vi "ArmFF_MaxAchieveVelocity.vi"(8 "Acceleration":dbl, 9 "Angle":dbl, 10 "MaxVoltage":dbl, 11 "in ARM_FF":T1 {"kCos" format="%13.5p"; "Ka" format="%13.5p"; "Kv" format="%13.5p"; "Ks" format="%13.5p"}) -> (3 "MaxVelocity":dbl)   [LabVIEW 2019, in "Trajectory_Library.lvlib"]
doc: "Calculates the maximum achievable velocity given a maximum voltage supply, a position, and an acceleration. Useful for ensuring that velocity and acceleration constraints for a trapezoidal profile are simultaneously achievable - enter the acceleration constraint, and this will give you a simultaneously-achievable velocity constraint.\n \nInputs: \n - ArmFF -- The ArmFF data cluster\n - maxVoltage -- The maximum voltage that can be supplied to the arm.\n - angle -- The angle of the arm. (radians)\n - acceleration -- The acceleration of the arm.\n\nOutputs:\n - MaxVelocity -- The maximum possible velocity at the given acceleration and angle."
uses:
  Trajectory_Library.lvlib
  ARM_FF.ctl
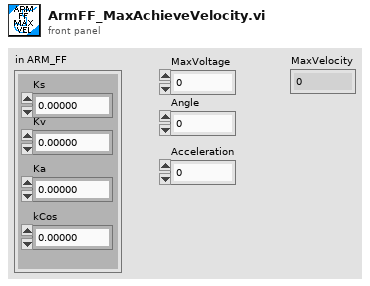
[diagram p1: front panel]
types:
  T1 = typedef "Trajectory_Library.lvlib/ARM_FF.ctl" = cluster{"Ks":dbl, "Kv":dbl, "Ka":dbl, "kCos":dbl}
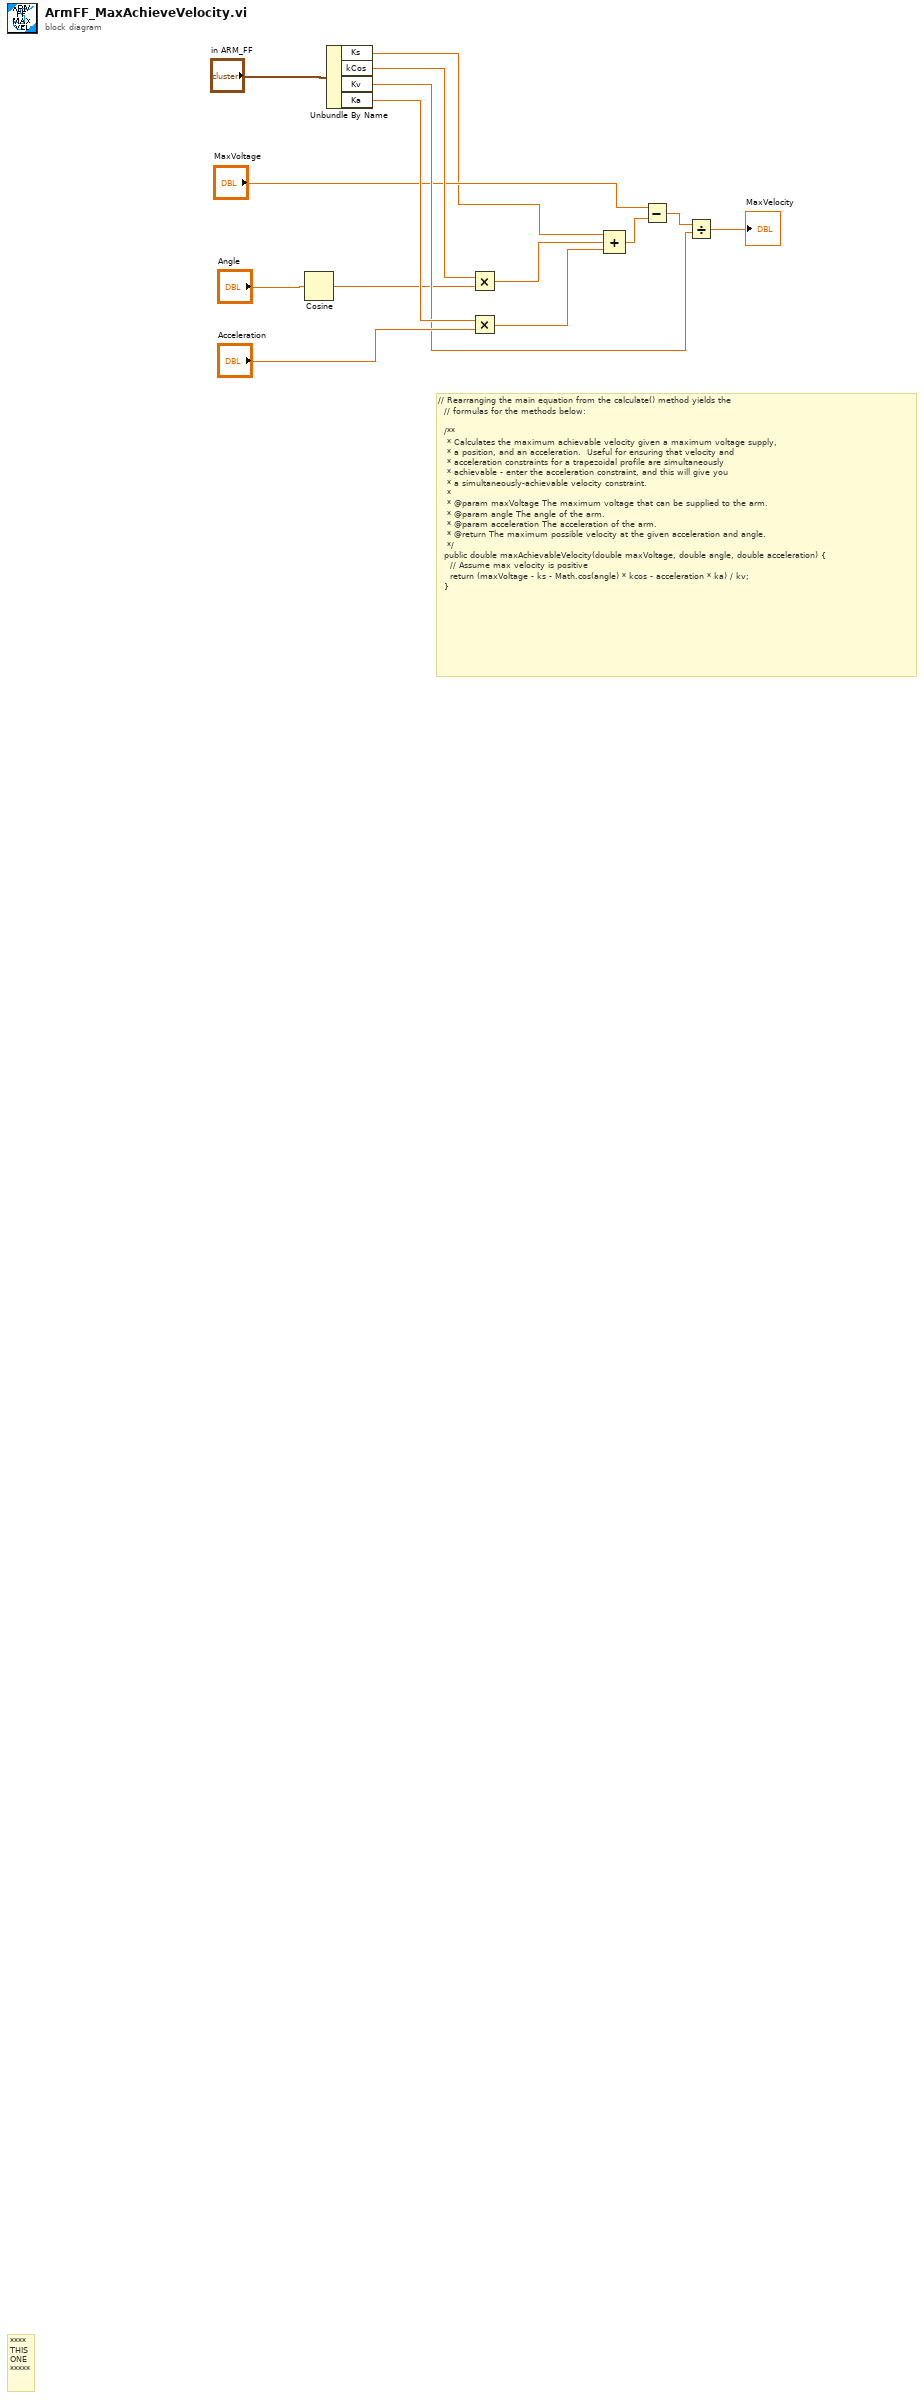
[diagram p0: block diagram]
diagram:
  # "// Rearranging the main equation from the calculate() method yields the\n  // formulas for the methods below:\n\n  /**\n   * Calculates the maximum achievable velocity given a maximum voltage supply,\n   * a position, and an acceleration.  Useful for ensuring that velocity and\n   * acceleration constraints for a trapezoidal profile are simultaneously\n   * achievable - enter the acceleration constraint, and this will give you\n   * a simultaneously-achievable velocity constraint.\n   *\n   * @param maxVoltage The maximum voltage that can be supplied to the arm.\n   * @param angle The angle of the arm.\n   * @param acceleration The acceleration of the arm.\n   * @return The maximum possible velocity at the given acceleration and angle.\n   */\n  public double maxAchievableVelocity(double maxVoltage, double angle, double acceleration) {\n    // Assume max velocity is positive\n    return (maxVoltage - ks - Math.cos(angle) * kcos - acceleration * ka) / kv;\n  }"
  # "****\nTHIS\nONE\n*****"
  n1 = Cosine(x="Angle") -> (cos(x)=w4:dbl)
  n2 = Unbundle By Name("in ARM_FF") -> ("Ks"=w3:dbl, "kCos"=w13:dbl, "Kv"=w9:dbl, "Ka"=w12:dbl)
  n3 = Multiply(x=w13, y=w4) -> (x*y=w2:dbl)
  n4 = Multiply(x=w12, y="Acceleration") -> (x*y=w1:dbl)
  n5 = Compound Arithmetic op=ADD(w3, w2, w1) -> (w7:dbl)
  n6 = Subtract(x="MaxVoltage", y=w7) -> (x-y=w8:dbl)
  n7 = Divide(x=w8, y=w9) -> (x/y=→"MaxVelocity":dbl)
